vi "Unpack for gRPC.vi"(8 "error in":errorcluster, 9 "configuration / results":enum16{"Configuration", "Results"}(ring), 10 "any":T1, 11 "measurement plugin in":refnum<class "CAN-LIN Frame Generator.lvclass">) -> (0 "error out":errorcluster, 2 "data value":variant, 3 "measurement plugin out":refnum<class "CAN-LIN Frame Generator.lvclass">)   [LabVIEW 2025, in "CAN-LIN Frame Generator.lvclass"]
uses:
  CAN-LIN Frame Generator.lvclass
  <vilib>/gRPC/LabVIEW gRPC Library/Shared/Any.ctl
  Measurement Configuration.ctl
  CAN-LIN Frame Generator UI/Toggle.ctl
  CAN-LIN Frame Generator UI/XNET Frame Type CAN.ctl
  Measurement Results.ctl
  a521b266-ce99-437c-923d-067dcf1e07fd.vi
  3ecd018e-d556-4cbc-bc60-c4ba57204520.vi
  <vilib>/gRPC/LabVIEW gRPC Library/Server API/Translate Protobuf Error.vi
  <vilib>/AdvancedString/1D String Array to Delimited String.vi
  <vilib>/gRPC/LabVIEW gRPC Library/Server API/Server/Get Server DLL Path.vi
  <vilib>/Plug-In SDKs/Measurements/Measurement Plugin Service/Measurement Plugin Service.lvclass
  <vilib>/gRPC/LabVIEW gRPC Library/grpc-lvsupport-release.lvlib
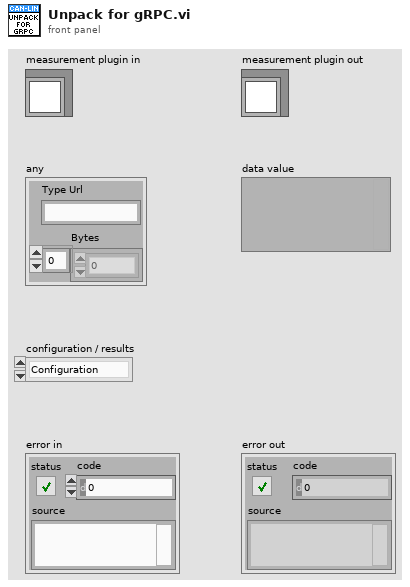
[diagram p1: front panel]
types:
  T1 = typedef "grpc-lvsupport-release.lvlib/Any.ctl" = cluster{"Type Url":string, "Bytes":u8[]}
  T2 = typedef "grpc-lvsupport-release.lvlib/grpcId.ctl" = u64
  T3 = typedef "CAN-LIN Frame Generator.lvclass/Measurement Configuration.ctl" = cluster{"INTERFACE NAME CAN":refnum<k21>, "IO Mode":enum32{"CAN", "CAN FD", "CAN FD + BRS"}, "FD ISO Mode":enum32{"ISO", "Legacy ISO", "Non-ISO"}, "Termination CAN":T4, "Baudrate":u32, "FD Baudrate":u32, "INTERFACE NAME LIN":refnum<k21>, "Termination LIN":T4, "CAN interface":string, "LIN interface":string, "IDENTIFIER":u32, "TYPE":T5, "DLC":u32, "SEND":bool, "IDENTIFIER 2":u32, "DLC 2":u32, "SEND 2":bool, "Tab No":string, "PAYLOAD":u32[], "PAYLOAD 2":u32[]}
  T4 = typedef "Toggle.ctl" = bool
  T5 = typedef "XNET Frame Type CAN.ctl" = u32
  T6 = typedef "CAN-LIN Frame Generator.lvclass/Measurement Results.ctl" = cluster{"DLC":u32, "DLC 2":u32}
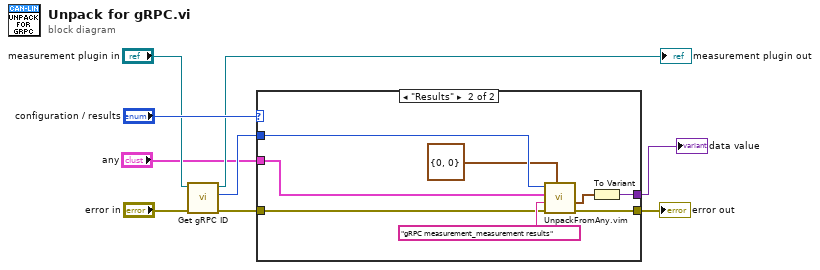
[diagram p0: block diagram]
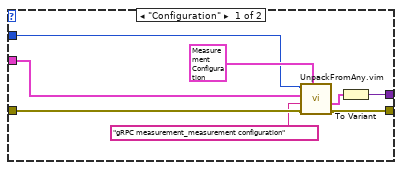
[diagram p2: hidden frame]
diagram:
  n1 = call <vilib>:"Get gRPC ID.vi"("error in"="error in", "measurement plugin service in"="measurement plugin in") -> ("error out"=w6:errorcluster, "gRPC ID"=w3:T2, "measurement plugin service out"=→"measurement plugin out":refnum<class "CAN-LIN Frame Generator.lvclass">)  [unwired: 7 in]
  n2 = case shown="\"Results\"" "configuration / results" {
    tunnel: w6 -> [w15 w19]
    tunnel: "any" -> [w10 w18]
    tunnel: w3 -> [w12 w22]
    tunnel: [w16 w23] -> w9
    tunnel: [w17 w25] -> w1
    frame "Configuration" {
      n3 = call "UnpackFromAny.vim"("Data Type"=T3 {"INTERFACE NAME CAN"="Lorem ipsum dolor sit", "IO Mode"=enum."CAN FD", "FD ISO Mode"=enum."Non-ISO", "Termination CAN"=TRUE, "Baudrate"=1, "FD Baudrate"=1, "INTERFACE NAME LIN"="", "Termination LIN"=FALSE, "CAN interface"="", "LIN interface"="", "IDENTIFIER"=4294967232, "TYPE"=0, "DLC"=0, "SEND"=FALSE, "IDENTIFIER 2"=0, "DLC 2"=0, "SEND 2"=FALSE, "Tab No"="", "PAYLOAD"=[], "PAYLOAD 2"=[0, 0]} ("Measurement Configuration"), "error in"=w15, "Message Type"="gRPC measurement_measurement configuration", "Any"=w10, "gRPCid in"=w12) -> ("error out"=w16:errorcluster, "Unpacked Value"=w14:T3)  [unwired: 4 in, 1 out]
      n4 = To Variant(anything=w14) -> (Variant=w17:variant)
    }
    frame "Results" {
      n5 = call "UnpackFromAny.vim"("Data Type"=T6 {"DLC"=0, "DLC 2"=0} ("Measurement Results"), "error in"=w19, "Message Type"="gRPC measurement_measurement results", "Any"=w18, "gRPCid in"=w22) -> ("error out"=w23:errorcluster, "Unpacked Value"=w24:T6)  [unwired: 4 in, 1 out]
      n6 = To Variant(anything=w24) -> (Variant=w25:variant)
    }
  }
  "error out" <- w9
  "data value" <- w1
